vi "定点周期设置.vi"(7 "Display State In":T1, 8 "测量参数字符串[]":string[](array[string]), 9 "间隔启动":T7, 10 "定点周期":T4, 11 "周期模式":T3) -> (2 "保存输出":bool, 3 "周期设置输出":T6)   [LabVIEW 2016, in "定时设置.xctl"]
panel:
  out "测试状态.结束时间":timestamp caption="结束时间" format="%<%y/%m/%d %H:%M:%S>T"
  out "测试状态.启动次数":dbl caption="启动次数"
  out "测试状态.启动时间":timestamp caption="启动时间" format="%<%y/%m/%d %H:%M:%S>T"
  in  "测量参数":T2
  in  "保存":bool
  in  "退出":bool
  in  "批量设置":bool
  out "周期模式选择卡":enum32{"选项卡 1", "选项卡 2"}(tab)
  # "分钟"
  # "次"
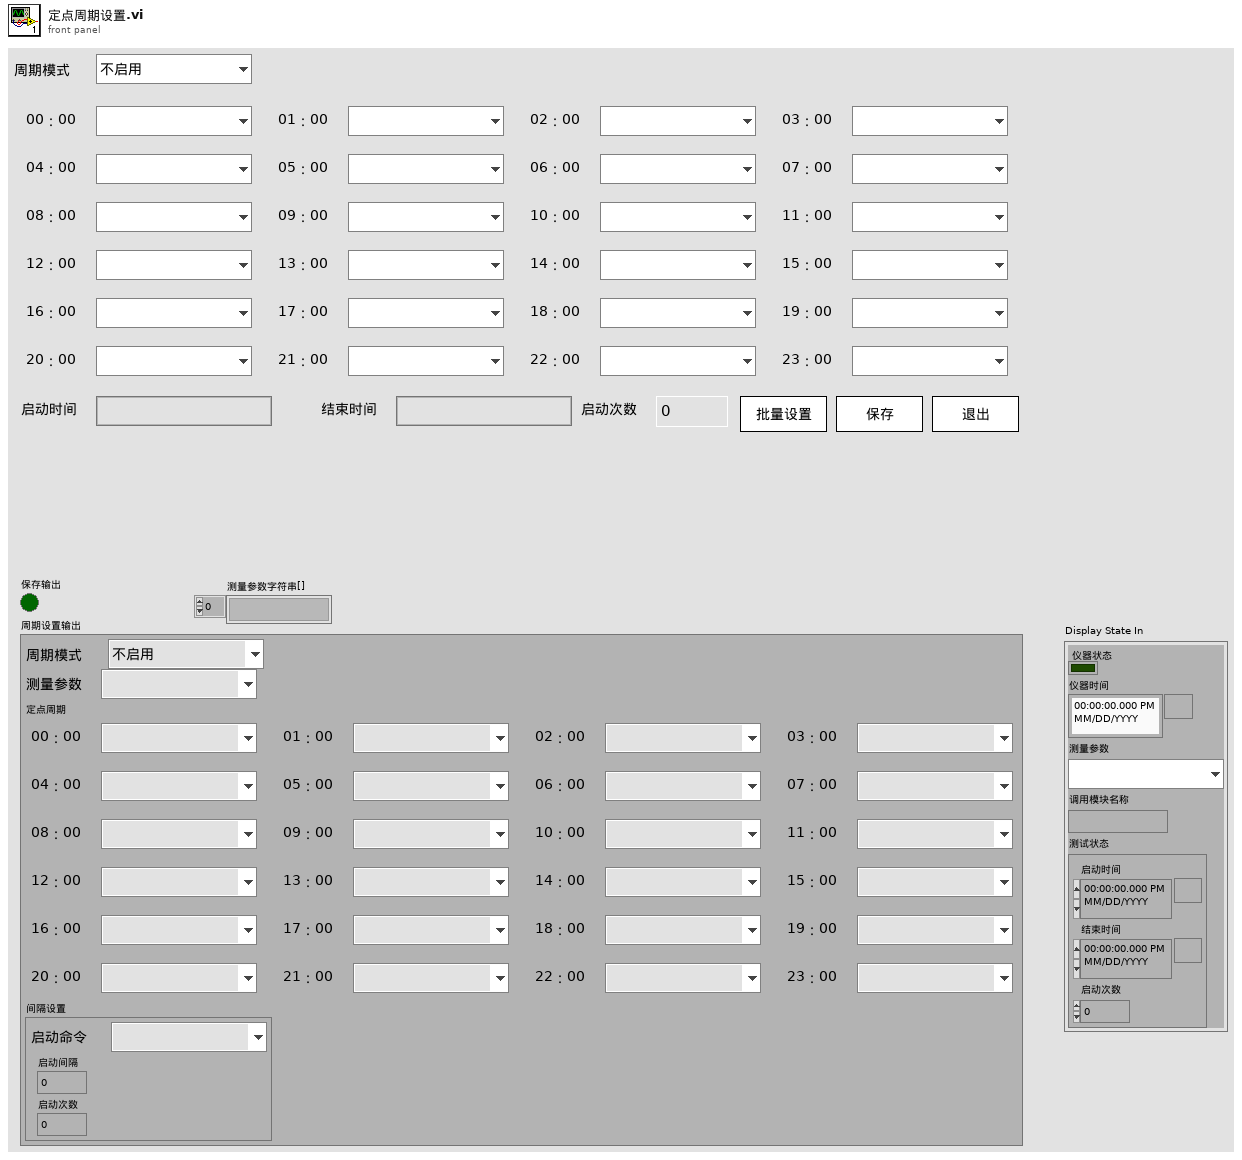
[diagram p1: front panel]
types:
  T1 = typedef "定时设置.xctl/状态 1.ctl" = cluster{"仪器状态":bool, "仪器时间":timestamp, "测量参数":T2, "调用模块名称":string, "测试状态":cluster{"启动时间":timestamp, "结束时间":timestamp, "启动次数":dbl}}
  T2 = typedef "定时设置.xctl/测量参数.ctl" = u16
  T3 = typedef "定时设置.xctl/周期模式设置.ctl" = enum16{"不启用", "定点模式", "间隔模式"}
  T4 = typedef "定时设置.xctl/定点周期设置.ctl" = cluster{"启动命令":T5, "启动命令 2":T5, "启动命令 3":T5, "启动命令 4":T5, "启动命令 5":T5, "启动命令 6":T5, "启动命令 7":T5, "启动命令 8":T5, "启动命令 9":T5, "启动命令 10":T5, "启动命令 11":T5, "启动命令 12":T5, "启动命令 13":T5, "启动命令 14":T5, "启动命令 15":T5, "启动命令 16":T5, "启动命令 17":T5, "启动命令 18":T5, "启动命令 19":T5, "启动命令 20":T5, "启动命令 21":T5, "启动命令 22":T5, "启动命令 23":T5, "启动命令 24":T5}
  T5 = typedef "定时设置.xctl/启动命令选择.ctl" = enum16{"", "水样测试", "标样核查", "零点核查", "跨度核查", "空白测试", "平行样测试", "加标回收", "空白校准", "标样校准"}
  T6 = cluster{"周期模式":T3, "测量参数":T2, "定点周期":T4, "间隔设置":cluster{"启动命令":T5, "启动间隔":dbl, "启动次数":i32}}
  T7 = typedef "定时设置.xctl/间隔启动设置.ctl" = cluster{"启动命令":T5, "启动间隔":dbl, "启动次数":i32}
  T8 = typedef "周期设置.lvlib/周期模式设置.ctl" = enum16{"不启用", "定点模式", "间隔模式"}
  T9 = cluster{"周期模式":T3, "测量参数":T2, "定点周期":T4, cluster{"启动命令":T5, "启动间隔":dbl, "启动次数":i32}}
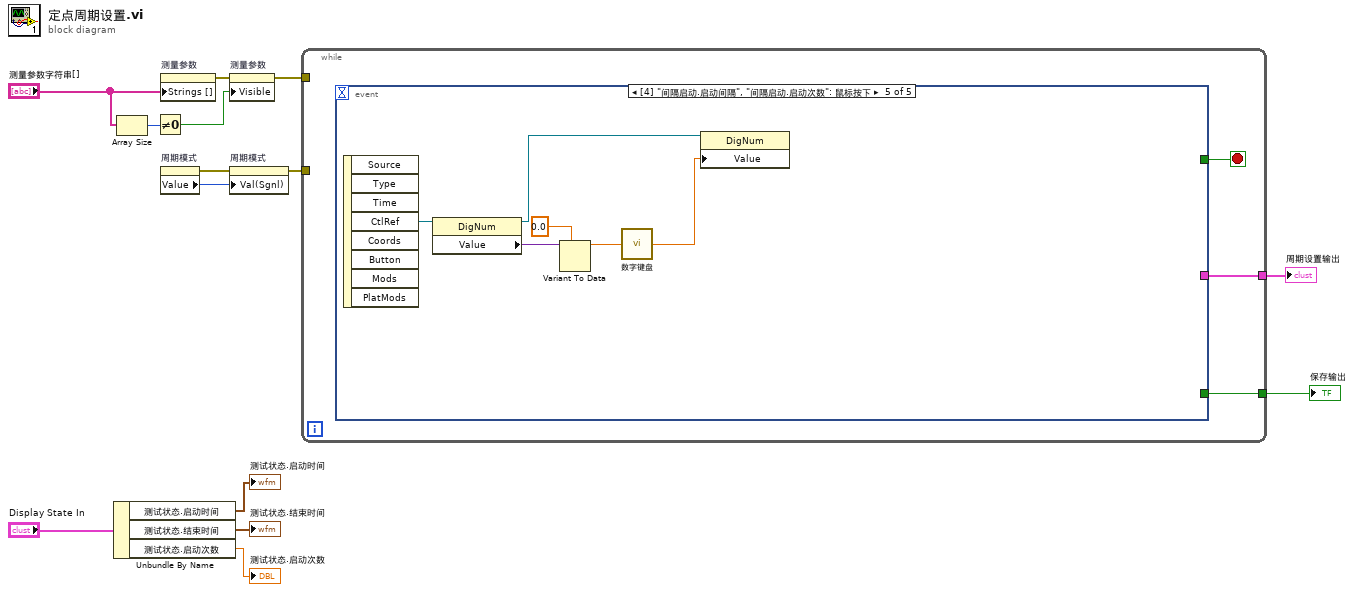
[diagram p0: block diagram]
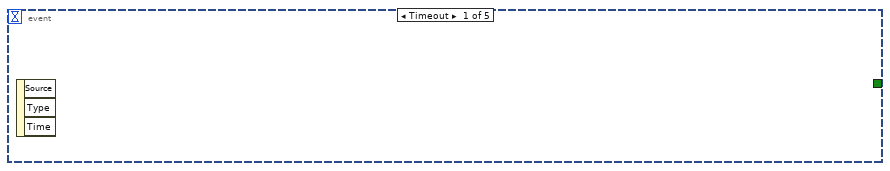
[diagram p2: hidden frame]
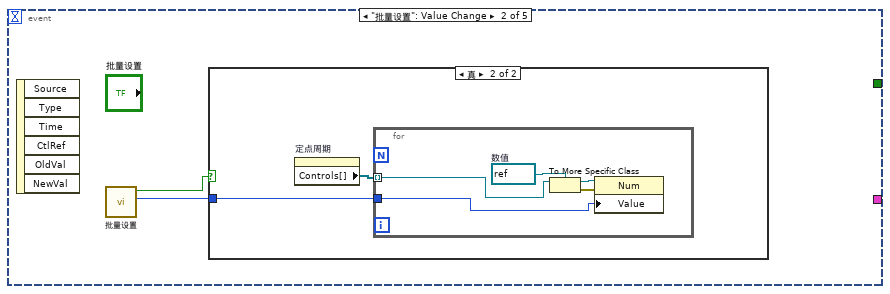
[diagram p3: hidden frame]
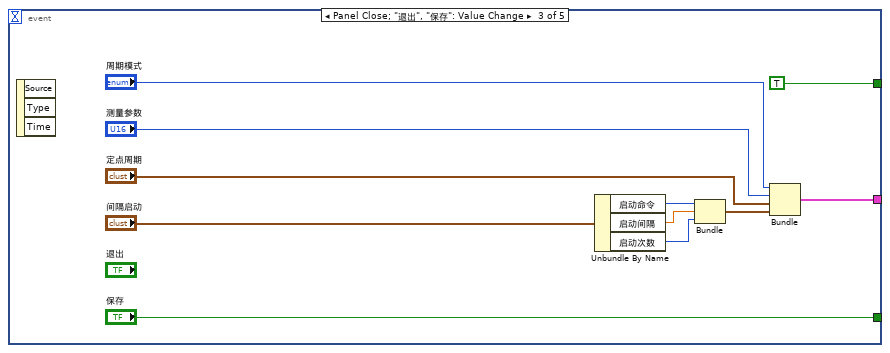
[diagram p5: hidden frame]
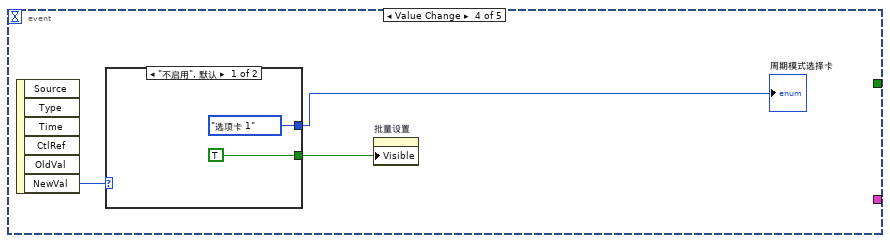
[diagram p6: hidden frame]
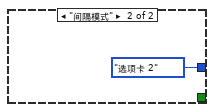
[diagram p7: hidden frame]
diagram:
  n1 = Unbundle By Name("Display State In") -> ("测试状态.启动时间"=→"测试状态.启动时间":timestamp, "测试状态.结束时间"=→"测试状态.结束时间":timestamp, "测试状态.启动次数"=→"测试状态.启动次数":dbl)
  n2 = Array Size(array="测量参数字符串[]") -> (size(s)=w5:i32)
  n3 = Not Equal To 0?(x=w5) -> (x != 0?=w8:bool)
  n4 = property on="测量参数" class="Ring (严格)"("Strings []"="测量参数字符串[]") -> (error out=w9:errorcluster)  [unwired: 2 in, 1 out]
  n5 = property on="周期模式" class="Enum (严格)"() -> (error out=w13:errorcluster, "Value"=w14:T8)  [unwired: 2 in, 1 out]
  n6 = property on="测量参数" class="Ring (严格)"(error in=w9, "Visible"=w8) -> (error out=w7:errorcluster)  [unwired: 1 in, 1 out]
  n7 = property on="周期模式" class="Enum (严格)"(error in=w13, "Val(Sgnl)"=w14) -> (error out=w12:errorcluster)  [unwired: 1 in, 1 out]
  n8 = while {
    tunnel: [w16] -> w11
    tunnel: w12 -> [_]
    tunnel: [w15] -> w10
    tunnel: w7 -> [_]
    stop <- w17 stop-if-true
    n9 = event shown="[4] \"间隔启动.启动间隔\", \"间隔启动.启动次数\": 鼠标按下" {
      selector: _ -> [_ _ _ _ _]
      dyn-events: _ -> [_ _ _ _ _]
      timeout: _ -> [_ _ _ _ _]
      tunnel: [_ _ TRUE _ _] -> w17
      tunnel: [_ _ w36 _ _] -> w16
      tunnel: [_ _ "保存" _ _] -> w15
      event Timeout {
        n10 = event-data() -> ()  [unwired: 1 in, 3 out]
      }
      event "批量设置": Value Change {
        n11 = event-data() -> ()  [unwired: 1 in, 6 out]
        n12 = call "批量设置.vi"() -> ("启动命令 2"=w19:T5, "确定 2"=w18:bool)  [unwired: 10 in]
        n13 = case shown="真" w18 {
          tunnel: w19 -> [_ w20]
          frame False {
          }
          frame True {
            n14 = property on="定点周期" class="Clust (严格)"() -> ("Controls[]"=w21:refnum<vi>[])  [unwired: 2 in, 2 out]
            n15 = for {
              tunnel: w21 -> [w26] mode=indexing
              tunnel: w20 -> [w22]
              w25 = refnum<vi> refnum  # 数值
              n16 = To More Specific Class(target class=w25, reference=w26) -> (specific class reference=w24:refnum<vi>, error out=w23:errorcluster)  [unwired: 1 in]
              n17 = property class="Num"(reference=w24, error in=w23, "Value"=w22) -> ()  [unwired: 2 out]
            }
          }
        }
      }
      event Panel Close; "退出", "保存": Value Change {
        n18 = event-data() -> ()  [unwired: 1 in, 3 out]
        n19 = Unbundle By Name("间隔启动") -> ("启动命令"=w33:T5, "启动间隔"=w32:dbl, "启动次数"=w31:i32)
        n20 = Bundle("启动命令"=w33, "启动间隔"=w32, "启动次数"=w31) -> (w30:cluster{"启动命令":T5, "启动间隔":dbl, "启动次数":i32})  [unwired: 1 in]
        n21 = Bundle("周期模式"="周期模式", "测量参数"="测量参数", "定点周期"="定点周期", w30) -> (w36:T9)  [unwired: 1 in]
      }
      event Value Change {
        n22 = event-data() -> ("NewVal"=w39:T3)  [unwired: 1 in, 5 out]
        n23 = case shown="\"不启用\", 默认" w39 {
          tunnel: [TRUE ("可见") _] -> w40
          tunnel: [enum32{"选项卡 1", "选项卡 2"}."选项卡 1" ("周期模式选择卡") enum32{"选项卡 1", "选项卡 2"}."选项卡 2" ("周期模式选择卡")] -> w38
          frame "不启用", Default {
          }
          frame "间隔模式" {
          }
        }
        "周期模式选择卡" <- w38
        n24 = property on="批量设置" class="Bool"("Visible"=w40) -> ()  [unwired: 2 in, 2 out]
      }
      event Mouse Down {
        n25 = event-data() -> ("CtlRef"=w49:refnum<vi>)  [unwired: 1 in, 7 out]
        n26 = property class="DigNum"(reference=w49) -> (reference out=w48:refnum<vi>, "Value"=w47:variant)  [unwired: 1 in, 1 out]
        n27 = Variant To Data(type=0.0, Variant=w47) -> (data=w45:dbl)  [unwired: 1 in, 1 out]
        n28 = call "数字键盘.vi"("OldNumber"=w45) -> ("NewNumber"=w44:sgl)
        n29 = property class="DigNum"(reference=w48, "Value"=w44) -> ()  [unwired: 1 in, 2 out]
      }
    }
  }
  "周期设置输出" <- w11
  "保存输出" <- w10
